vi "RelTurn.vi"(11 "Angle":dbl) -> ()   [LabVIEW 2015]
uses:
  <vilib>/Rock Robotics/Network Tables/NT Read Number.vi
  <vilib>/Rock Robotics/Network Tables/NT Write Boolean.vi
  <vilib>/Rock Robotics/Network Tables/NT Write Number.vi
  <vilib>/addons/control/pid/pid.llb/PID (DBL).vi
  NavX/navX Library v2/navX Library v2.lvlib
  <vilib>/addons/control/pid/NI_PID_pid.lvlib
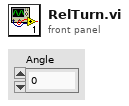
[diagram p1: front panel]
types:
  T1 = typedef "navX Library v2.lvlib/Z900_navX_DeviceTypeDef.ctl" = cluster{"Interface":cluster{"Protocol":T2, "Update Rate (4Hz-60Hz)":u8, "navX Open TypeDef":variant}, "Notify Packet":refnum<notifier>, "Loop VI Refnum":refnum<vi>, "Ready to Close Occurrence Refnum":refnum<k4>}
  T2 = typedef "navX Library v2.lvlib/Z900_navX_ProtocolTypeDef.ctl" = enum16{"SERIAL", "I2C", "SPI"}
  T3 = cluster{"Yaw":dbl, "Roll":dbl, "Pitch":dbl, "Heading":dbl, "Fused Heading":dbl}
  T4 = cluster{"Accel X":dbl, "Accel Y":dbl, "Accel Z":dbl, "Gyro X":dbl, "Gyro Y":dbl, "Gyro Z":dbl, "Mag X":dbl, "Mag Y":dbl, "Mag Z":dbl}
  T5 = cluster{"Numeric":dbl, "Numeric":dbl, "Numeric":dbl}
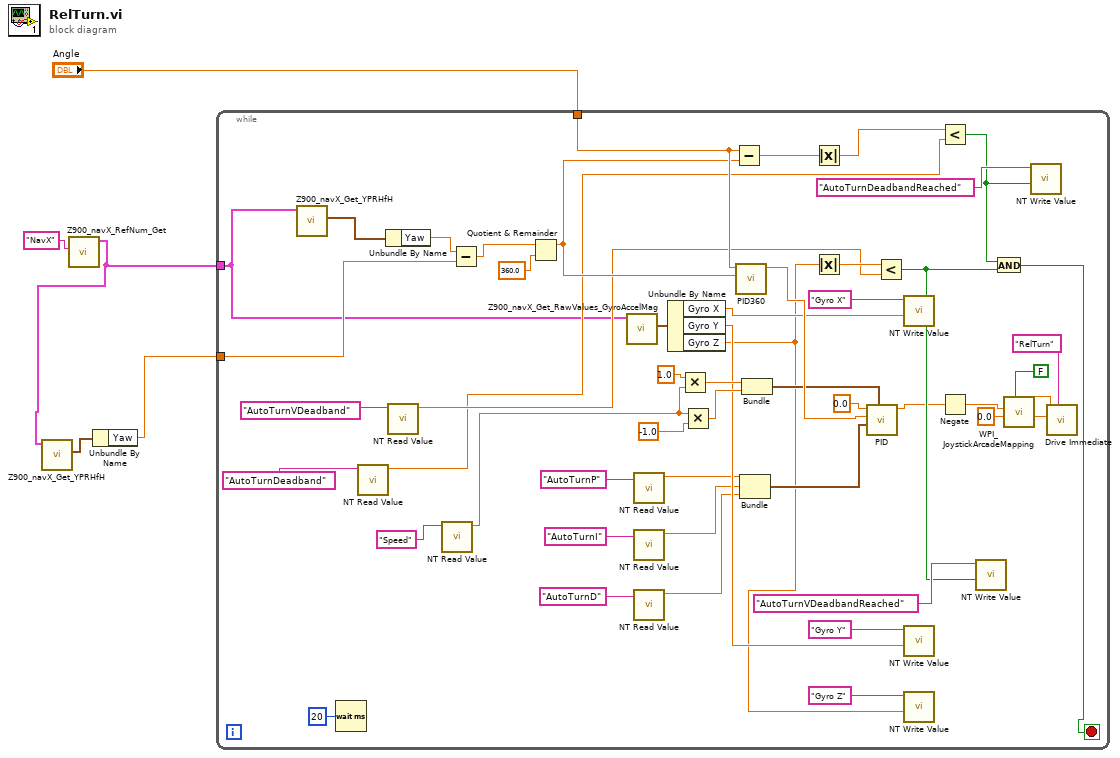
[diagram p0: block diagram]
diagram:
  n1 = call "Z900_navX_RefNum_Get.vi"("refnum name"="NavX") -> ("navX Device"=w1:T1)  [unwired: 9 in, 1 out]
  n2 = call "Z900_navX_Get_YPRHfH.vi"("navX Device"=w1) -> ("YRPHfH"=w2:T3)  [unwired: 7 in, 3 out]
  n3 = Unbundle By Name(w2) -> ("Yaw"=w5:dbl)
  n4 = while {
    tunnel: w1 -> [w13]
    tunnel: w5 -> [w53]
    tunnel: "Angle" -> [w31]
    stop <- w17 stop-if-true
    n5 = call "Z900_navX_Get_YPRHfH.vi"("navX Device"=w13) -> ("YRPHfH"=w15:T3)  [unwired: 7 in, 3 out]
    n6 = Wait (ms)(milliseconds to wait=u32 20) -> ()  [unwired: 1 out]
    n7 = call-poly <vilib>:"NT Read Value.vi"("Name"="AutoTurnDeadband") -> ("Numeric"=w18:dbl)  [unwired: 9 in, 1 out]
    n8 = Unbundle By Name(w15) -> ("Yaw"=w54:dbl)
    n9 = call-poly <vilib>:"NT Read Value.vi"("Name"="AutoTurnVDeadband") -> ("Numeric"=w19:dbl)  [unwired: 9 in, 1 out]
    n10 = call-poly <vilib>:"NT Read Value.vi"("Name"="Speed") -> ("Numeric"=w22:dbl)  [unwired: 9 in, 1 out]
    n11 = Subtract(x=w54, y=w53) -> (x-y=w55:dbl)
    n12 = Quotient & Remainder(x=w55, y=360.0) -> (x-y*floor(x/y)=w30:dbl)  [unwired: 1 out]
    n13 = call "Z900_navX_Get_RawValues_GyroAccelMag.vi"("navX Device"=w13) -> ("Raw Values"=w14:T4)  [unwired: 7 in, 3 out]
    n14 = call-poly <vilib>:"NT Read Value.vi"("Name"="AutoTurnP") -> ("Numeric"=w26:dbl)  [unwired: 9 in, 1 out]
    n15 = call-poly <vilib>:"NT Read Value.vi"("Name"="AutoTurnI") -> ("Numeric"=w24:dbl)  [unwired: 9 in, 1 out]
    n16 = call-poly <vilib>:"NT Read Value.vi"("Name"="AutoTurnD") -> ("Numeric"=w25:dbl)  [unwired: 9 in, 1 out]
    n17 = Unbundle By Name(w14) -> ("Gyro X"=w42:dbl, "Gyro Y"=w41:dbl, "Gyro Z"=w37:dbl)
    n18 = Multiply(x=1.0, y=w22) -> (x*y=w47:dbl)
    n19 = Multiply(x=w22, y=-1.0) -> (x*y=w48:dbl)
    n20 = Subtract(x=w31, y=w30) -> (x-y=w44:dbl)
    n21 = call "PID360.vi"("Robot"=w30, "Target"=w31) -> ("Numeric"=w52:dbl)  [unwired: 9 in]
    n22 = Bundle("Numeric"=w26, "Numeric"=w24, "Numeric"=w25) -> (w45:T5)  [unwired: 1 in]
    n23 = Bundle(w47, w48) -> (w46:cluster{dbl, dbl})  [unwired: 1 in]
    n24 = Absolute Value(x=w44) -> (abs(x)=w43:dbl)
    n25 = Absolute Value(x=w37) -> (abs(x)=w36:dbl)
    n26 = call-poly <vilib>:"PID.vi"("output range"=w46, "PID gains"=w45, "process variable"=w52, "setpoint"=0.0) -> ("output"=w7:dbl)  [unwired: 6 in, 1 out]
    n27 = Less?(x=w36, y=w19) -> (x < y?=w33:bool)
    n28 = call-poly <vilib>:"NT Write Value.vi"("Numeric"=w42, "Name"="Gyro X") -> ()  [unwired: 9 in, 1 out]
    n29 = call-poly <vilib>:"NT Write Value.vi"("Numeric"=w41, "Name"="Gyro Y") -> ()  [unwired: 9 in, 1 out]
    n30 = call-poly <vilib>:"NT Write Value.vi"("Numeric"=w37, "Name"="Gyro Z") -> ()  [unwired: 9 in, 1 out]
    n31 = Less?(x=w43, y=w18) -> (x < y?=w32:bool)
    n32 = Negate(x=w7) -> (-x=w6:dbl)
    n33 = call-poly <vilib>:"NT Write Value.vi"("Boolean"=w33, "Name"="AutoTurnVDeadbandReached") -> ()  [unwired: 9 in, 1 out]
    n34 = And(x=w32, y=w33) -> (x .and. y?=w17:bool)
    n35 = call <vilib>:"WPI_JoystickArcadeMapping.vi"("Square Inputs"=FALSE, "Y axis value"=0.0, "X axis value"=w6) -> ("Right Motor Value"=w10:dbl, "Left Motor Value"=w9:dbl)  [unwired: 7 in]
    n36 = call-poly <vilib>:"NT Write Value.vi"("Boolean"=w32, "Name"="AutoTurnDeadbandReached") -> ()  [unwired: 9 in, 1 out]
    n37 = call "Drive Immediate.vi"("Description"="RelTurn", "Right Setpoint"=w10, "Left Setpoint"=w9) -> ()  [unwired: 8 in, 1 out]
  }
